vi "Serial_WrRd_Array.vi"(6 "Read Delay (ms)":u16 max=5000 step=100, 9 "WR Size":u16 step=1, 10 "Array":u8[](array[numeric]) format="%x", 11 "ComPort":refnum<visa-resource-name>="COM10") -> (0 "error out":errorcluster, 2 "read butes row":u8[](array[numeric]), 3 "received":string)   [LabVIEW 2018]
uses:
  <vilib>/Instr/_visa.llb/VISA Configure Serial Port (Instr).vi
panel:
  out "read buf row":string
  # "ADB Serial W/R Array"
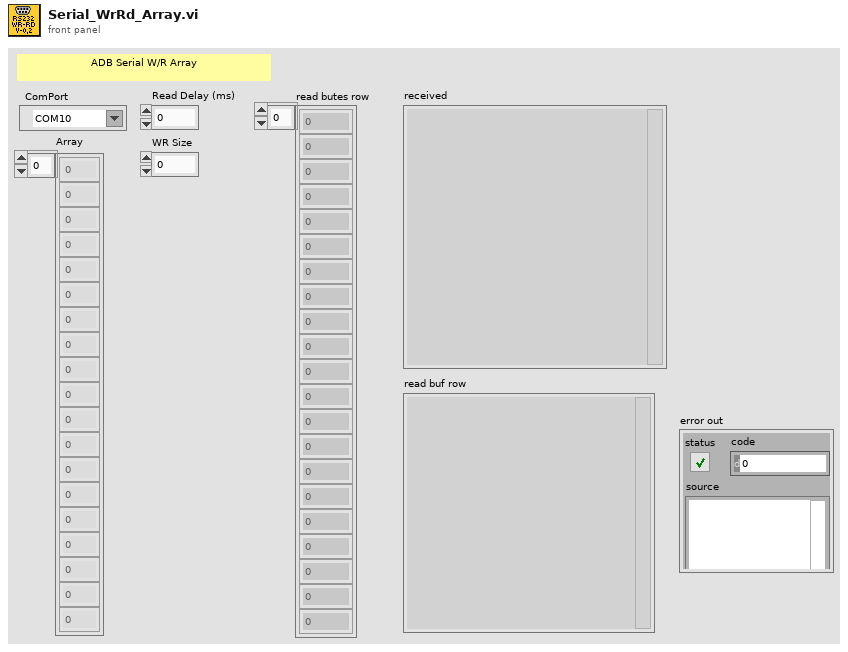
[diagram p1: front panel]
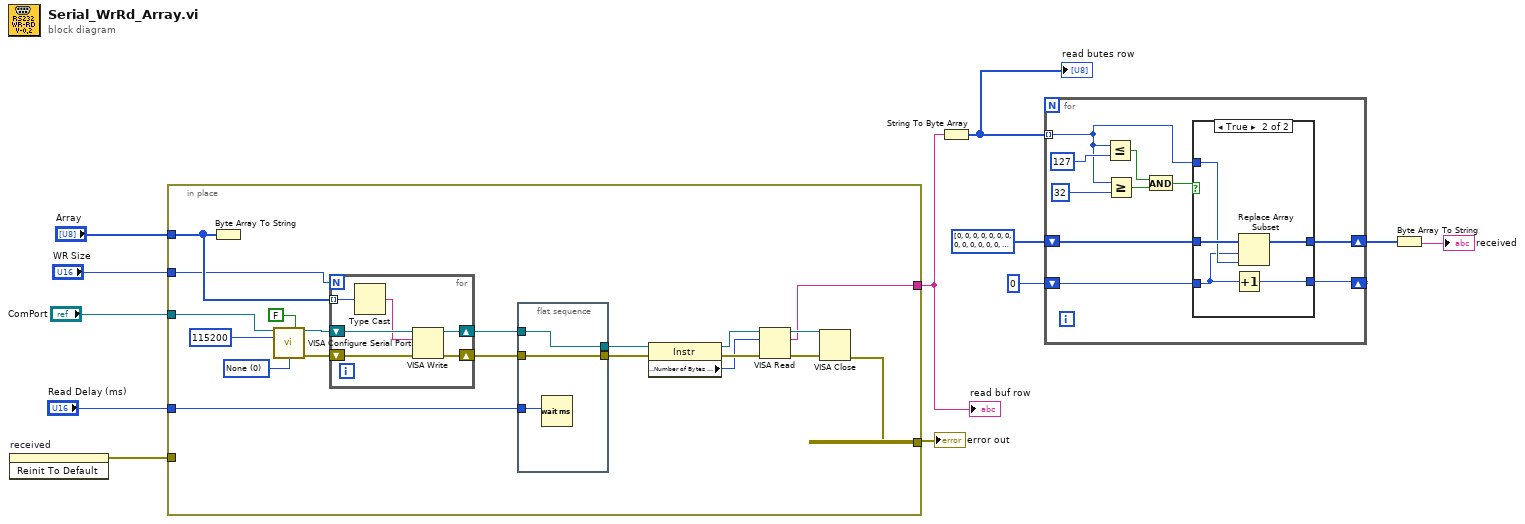
[diagram p0: block diagram]
diagram:
  n1 = invoke on="received" class="Str" method="Reinit To Default"() -> (error out=w11:errorcluster)  [unwired: 3 in, 2 out]
  n2 = in-place {
    in-place-border: "ComPort" -> [w32]
    in-place-border: [w31] -> w8
    in-place-border: [w20] -> w6
    in-place-border: w11 -> [_]
    in-place-border: "Array" -> [w14]
    in-place-border: "Read Delay (ms)" -> [w15]
    in-place-border: "WR Size" -> [w13]
    w21 = u16 0 items=["None", "XON/XOFF", "RTS/CTS", "XON/XOFF & RTS/CTS", "DTR/DSR", "XON/XOFF & DTR/DSR"] ("flow control (0:none)")
    n3 = Byte Array To String(unsigned byte array=w14) -> ()  [unwired: 1 out]
    n4 = call-poly "VISA Configure Serial Port"("VISA resource name"=w32, "Enable Termination\nChar (T)"=FALSE ("Enable Termination\nChar (T)"), "baud rate (9600)"=u32 115200 ("Serial Settings:Baud Rate"), "flow control (0:none)"=w21) -> ("VISA resource name out"=w30:refnum<visa-resource-name>, "error out"=w29:errorcluster)  [unwired: 10 in]
    n5 = for {
      N: w13 -> [_]
      shift-right: [w35] -> w16
      shift-left: w30 -> [w38]
      shift-right: [w36] -> w18
      shift-left: w29 -> [w37]
      tunnel: w14 -> [w34] mode=indexing
      n6 = Type Cast(x=w34) -> (*(type *) &x=w33:string)  [unwired: 1 in]
      n7 = VISA Write(VISA resource name=w38, write buffer=w33, error in (no error)=w37) -> (VISA resource name out=w35:refnum<visa-resource-name>, error out=w36:errorcluster)  [unwired: 1 out]
    }
    n8 = flat-sequence {
      tunnel: [w41] -> w19
      tunnel: w18 -> [w41]
      tunnel: [w40] -> w17
      tunnel: w16 -> [w40]
      tunnel: w15 -> [w39]
      frame #0 {
        n9 = Wait (ms)(milliseconds to wait=w39) -> ()  [unwired: 1 out]
      }
    }
    n10 = property class="Instr"(reference=w17, error in=w19) -> (reference out=w25:refnum<visa-resource-name>, error out=w26:errorcluster, "Serial Settings:Number of Bytes at Serial Port"=w24:u32)
    n11 = VISA Read(VISA resource name=w25, byte count=w24, error in (no error)=w26) -> (VISA resource name out=w28:refnum<visa-resource-name>, read buffer=w20:string, error out=w27:errorcluster)  [unwired: 1 out]
    n12 = VISA Close(VISA resource name=w28, error in (no error)=w27) -> (error out=w31:errorcluster)
  }
  "error out" <- w8
  "read buf row" <- w6
  n13 = String To Byte Array(string=w6) -> (unsigned byte array=w5:u8[])
  "read butes row" <- w5
  n14 = for {
    tunnel: w5 -> [w44] mode=indexing
    shift-right: [w49] -> w3
    shift-left: u8[] [0, 0, 0, 0, 0, 0, 0, 0, 0, 0, 0, 0, 0, 0, 0, 0, 0, 0, 0, 0, 0, 0, 0, 0, 0, 0, 0, 0, 0, 0, 0, 0, 0, 0, 0, 0, 0, 0, 0, 0, 0, 0, 0, 0, 0, 0, 0, 0, 0, 0, 0, 0, 0, 0, 0, 0, 0, 0, 0, 0, 0, 0, 0, 0, 0, 0, 0, 0, 0, 0, 0, 0, 0, 0, 0, 0, 0, 0, 0, 0, 0, 0, 0, 0, 0, 0, 0, 0, 0, 0, 0, 0, 0, 0, 0, 0, 0, 0, 0, 0, 0, 0, 0, 0, 0, 0, 0, 0, 0, 0, 0, 0, 0, 0, 0, 0, 0, 0, 0, 0, 0, 0, 0, 0, 0, 0, 0, 0, 0, 0, 0, 0, 0, 0, 0, 0, 0, 0, 0, 0, 0, 0, 0, 0, 0, 0, 0, 0, 0, 0, 0, 0, 0, 0, 0, 0, 0, 0, 0, 0, 0, 0, 0, 0, 0, 0, 0, 0, 0, 0, 0, 0, 0, 0, 0, 0, 0, 0, 0, 0, 0, 0, 0, 0, 0, 0, 0, 0, 0, 0, 0, 0, 0, 0, 0, 0, 0, 0, 0, 0, 0, 0, 0, 0, 0, 0, 0, 0, 0, 0, 0, 0, 0, 0, 0, 0, 0, 0, 0, 0, 0, 0, 0, 0, 0, 0, 0, 0, 0, 0, 0, 0, 0, 0, 0, 0, 0, 0, 0, 0, 0, 0, 0, 0, 0, 0, 0, 0, 0, 0, 0, 0, 0, 0, 0, 0] -> [w50]
    shift-right: [w42] -> _
    shift-left: 0 -> [w43]
    n15 = Less Or Equal?(x=w44, y=127) -> (x <= y?=w47:bool)
    n16 = Greater Or Equal?(x=w44, y=u8 32) -> (x >= y?=w46:bool)
    n17 = And(x=w47, y=w46) -> (x .and. y?=w45:bool)
    n18 = case shown="True" w45 {
      tunnel: w44 -> [_ w56]
      tunnel: w50 -> [w53 w57]
      tunnel: [w53 w58] -> w49
      tunnel: w43 -> [w52 w55]
      tunnel: [w52 w54] -> w42
      frame False {
      }
      frame True {
        n19 = Increment(x=w55) -> (x+1=w54:i32)
        n20 = Replace Array Subset(array=w57, new element=w56, index=w55) -> (w58:u8[])
      }
    }
  }
  n21 = Byte Array To String(unsigned byte array=w3) -> (string=→"received":string)
